vi "move_tilt_stage_simpler(Sub VI).vi"(4 ".NET Refnum in":refnum<k24>, 5 "error in (no error)":errorcluster, 6 "motor":i32, 7 "relativeSteps":i32, 8 "deviceKey":string) -> (0 "error out":errorcluster, 1 "End position":i32, 2 "Initial position":i32, 3 ".NET Refnum out":refnum<k24>)   [LabVIEW 2016]
uses:
  C:/Users/UsphereLab/Documents/GitHub/Optlev/LabView Code/Examples/Tilt Stage/CmdLib.dll
  Examples/Tilt Stage/CmdLib.dll
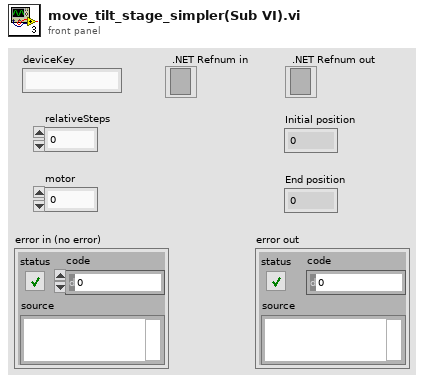
[diagram p1: front panel]
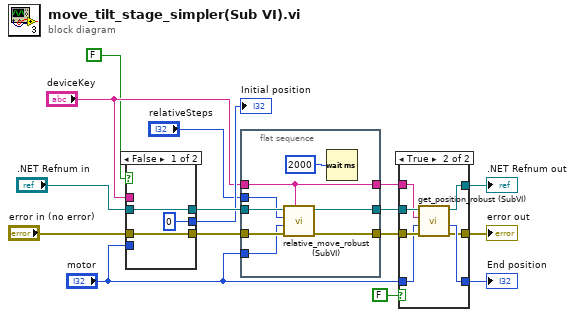
[diagram p0: block diagram]
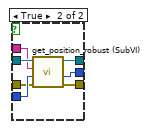
[diagram p2: hidden frame]
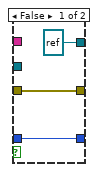
[diagram p3: hidden frame]
diagram:
  n1 = case shown="False" FALSE {
    tunnel: [w18 w26] -> w14
    tunnel: [w19 w25] -> w13
    tunnel: "motor" -> [_ w24]
    tunnel: [0 ("position") w23] -> w11
    tunnel: ".NET Refnum in" -> [w18 w22]
    tunnel: "deviceKey" -> [_ w21]
    tunnel: "error in (no error)" -> [w19 w20]
    frame False {
    }
    frame True {
      n2 = call "get_position_robust (SubVI).vi"("error in (no error)"=w20, "motor"=w24, "deviceKey"=w21, ".NET Refnum in"=w22) -> ("error out"=w25:errorcluster, "position"=w23:i32, ".NET Refnum out"=w26:refnum<k24>)  [unwired: 4 in, 1 out]
    }
  }
  "Initial position" <- w11
  n3 = flat-sequence {
    tunnel: w14 -> [w34]
    tunnel: "relativeSteps" -> [w33]
    tunnel: w13 -> [w32]
    tunnel: "motor" -> [w31]
    tunnel: "deviceKey" -> [w28]
    tunnel: [w30] -> w16
    tunnel: [w29] -> w15
    tunnel: [w28] -> w10
    frame #0 {
      n4 = call "relative_move_robust (SubVI).vi"("deviceKey"=w28, "error in (no error)"=w32, "motor"=w31, "relativeSteps"=w33, ".NET Refnum in"=w34) -> ("error out"=w29:errorcluster, ".NET Refnum out"=w30:refnum<k24>)  [unwired: 5 in]
      n5 = Wait (ms)(milliseconds to wait=u32 2000) -> ()  [unwired: 1 out]
    }
  }
  n6 = case shown="True" FALSE {
    tunnel: w16 -> [_ w44]
    tunnel: w15 -> [w37 w43]
    tunnel: [w36 w42] -> w1
    tunnel: "motor" -> [w36 w41]
    tunnel: w10 -> [_ w40]
    tunnel: [w37 w39] -> w9
    tunnel: [refnum<k24> refnum (".NET Refnum out") w38] -> w2
    frame False {
    }
    frame True {
      n7 = call "get_position_robust (SubVI).vi"("error in (no error)"=w43, "motor"=w41, "deviceKey"=w40, ".NET Refnum in"=w44) -> ("error out"=w39:errorcluster, "position"=w42:i32, ".NET Refnum out"=w38:refnum<k24>)  [unwired: 4 in, 1 out]
    }
  }
  "error out" <- w9
  "End position" <- w1
  ".NET Refnum out" <- w2
